vi "Read Path.vi"(7 "key":string, 8 "error in (no error)":errorcluster, 9 "default value":path, 11 "Configuration In":refnum<class "Configuration.lvclass">) -> (0 "error out":errorcluster, 1 "value":path, 3 "Configuration Out":refnum<class "Configuration.lvclass">)   [LabVIEW 2020, in "Astemes_CSVReportPlugin.lvlib" / "Configuration.lvclass"]
doc: "High-level function for reading configuration file data from process class. If the specified key is not present, it is added with the configured default value."
uses:
  Configuration.lvclass
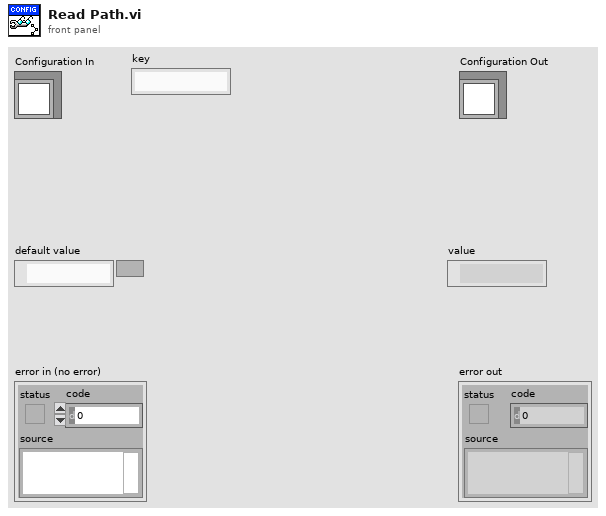
[diagram p1: front panel]
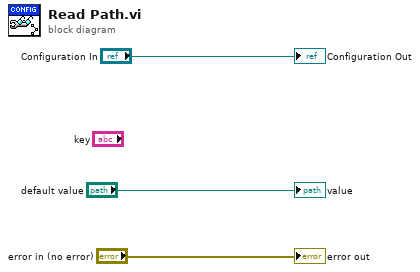
[diagram p0: block diagram]
diagram:
  "error out" <- "error in (no error)"
  "Configuration Out" <- "Configuration In"
  "value" <- "default value"
